vi "Open File on Disk.vi"(8 "error in":errorcluster, 11 "file or directory path":path) -> (0 "error out":errorcluster)   [LabVIEW 2020, in "Panther Dashboard.lvlib"]
uses:
  Panther Dashboard.lvlib
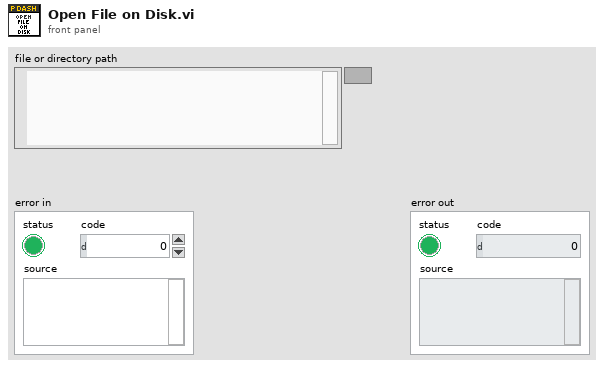
[diagram p1: front panel]
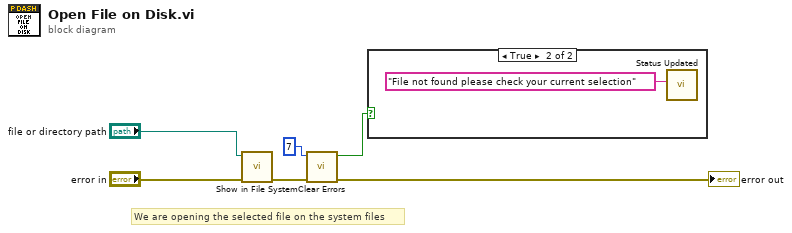
[diagram p0: block diagram]
diagram:
  # "We are opening the selected file on the system files"
  n1 = call <vilib>:"Show in File System.vi"("error in (no error)"="error in", "file or directory path"="file or directory path") -> ("error out"=w4:errorcluster)  [unwired: 9 in]
  n2 = call <vilib>:"Clear Errors.vi"("error in (no error)"=w4, "specific error code to clear (0: all)"=7) -> ("error out"=→"error out":errorcluster, "specific error cleared?"=w1:bool)  [unwired: 4 in]
  n3 = case shown="True" w1 {
    frame False {
    }
    frame True {
      n4 = call "Status Updated.vi"("Status"="File not found please check your current selection") -> ()  [unwired: 10 in, 1 out]
    }
  }
